vi "Verify Checksum.vi"(1 "HEX String to Verify CheckSum":string) -> (0 "CheckSum OK":bool)   [LabVIEW 2014]
panel:
  out "Message Length":dbl
  out "Total Message Length":dbl
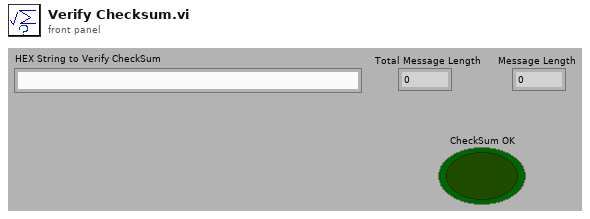
[diagram p1: front panel]
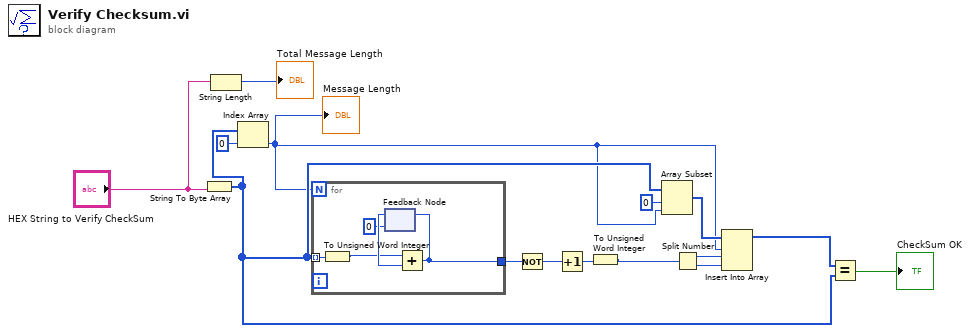
[diagram p0: block diagram]
diagram:
  n1 = String To Byte Array(string="HEX String to Verify CheckSum") -> (unsigned byte array=w3:u8[])
  n2 = String Length(string="HEX String to Verify CheckSum") -> (length=→"Total Message Length":i32)
  n3 = Index Array(array=w3, index=0) -> (element=w1:u8)
  "Message Length" <- w1
  n4 = for {
    N: w1 -> [_]
    tunnel: w3 -> [w16] mode=indexing
    tunnel: [w19] -> w15
    n5 = To Unsigned Word Integer(number=w16) -> (unsigned 16bit integer=w17:u16)
    n6 = feedback #1(u8 0) -> (w20:u8)
    n7 = Add(x=w17, y=w20) -> (x+y=w19:u16)
    n8 = feedback-in #1(w19) -> ()
  }
  n9 = Not(x=w15) -> (.not. x?=w14:u16)
  n10 = Increment(x=w14) -> (x+1=w11:u16)
  n11 = To Unsigned Word Integer(number=w11) -> (unsigned 16bit integer=w10:u16)
  n12 = Array Subset(array=w3, index=0, length=w1) -> (w4:u8[])
  n13 = Split Number(x=w10) -> (hi(x)=w13:u8, lo(x)=w12:u8)
  n14 = Insert Into Array(array=w4, index=w1, new element #1=w13, new element #2=w12) -> (w7:u8[])
  n15 = Equal?(x=w7, y=w3) -> (x = y?=→"CheckSum OK":bool)
